vi "2B_Tech_TCP_Packet_TWBOZO_v1.vi"(7 "TCP Packet In":string, 12 "Data Array":string[](array[string])) -> (8 "TCP Binary Packet":string)   [LabVIEW 2014]
panel:
  out "array":string[](array[string])
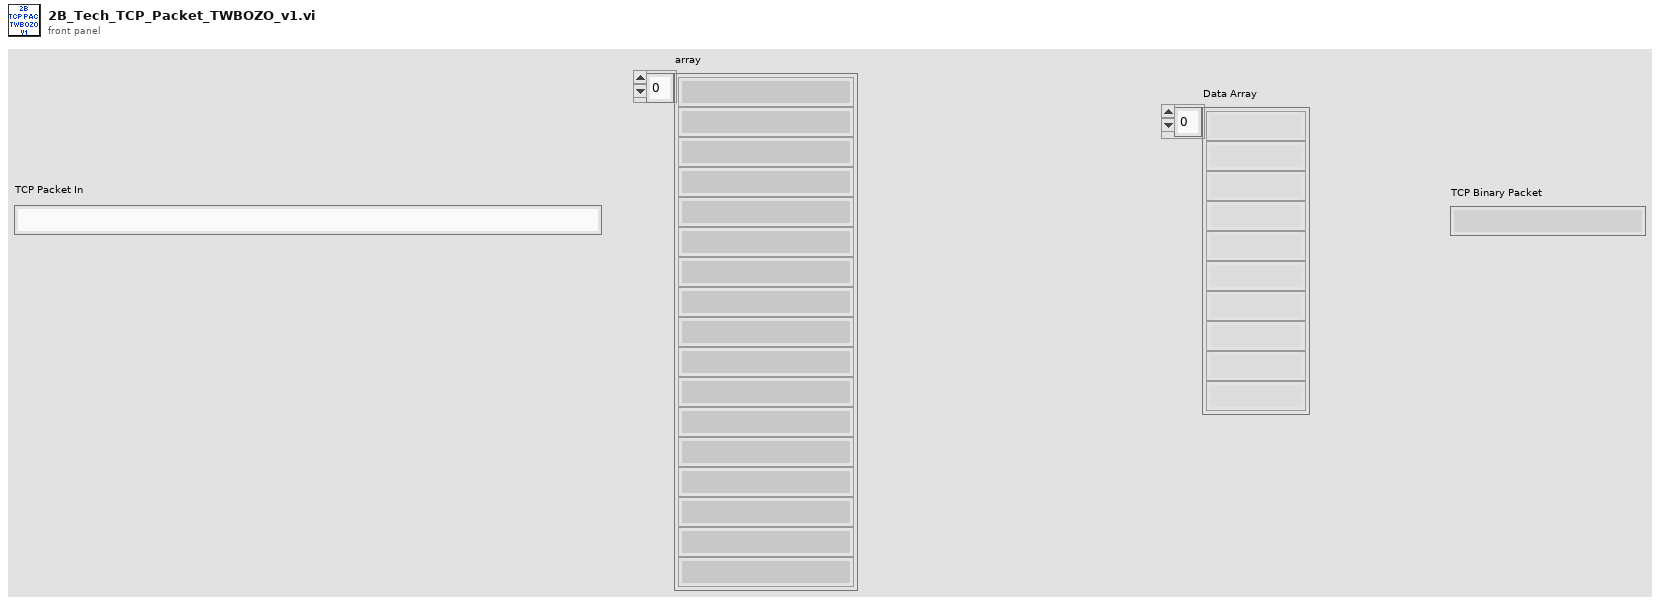
[diagram p1: front panel]
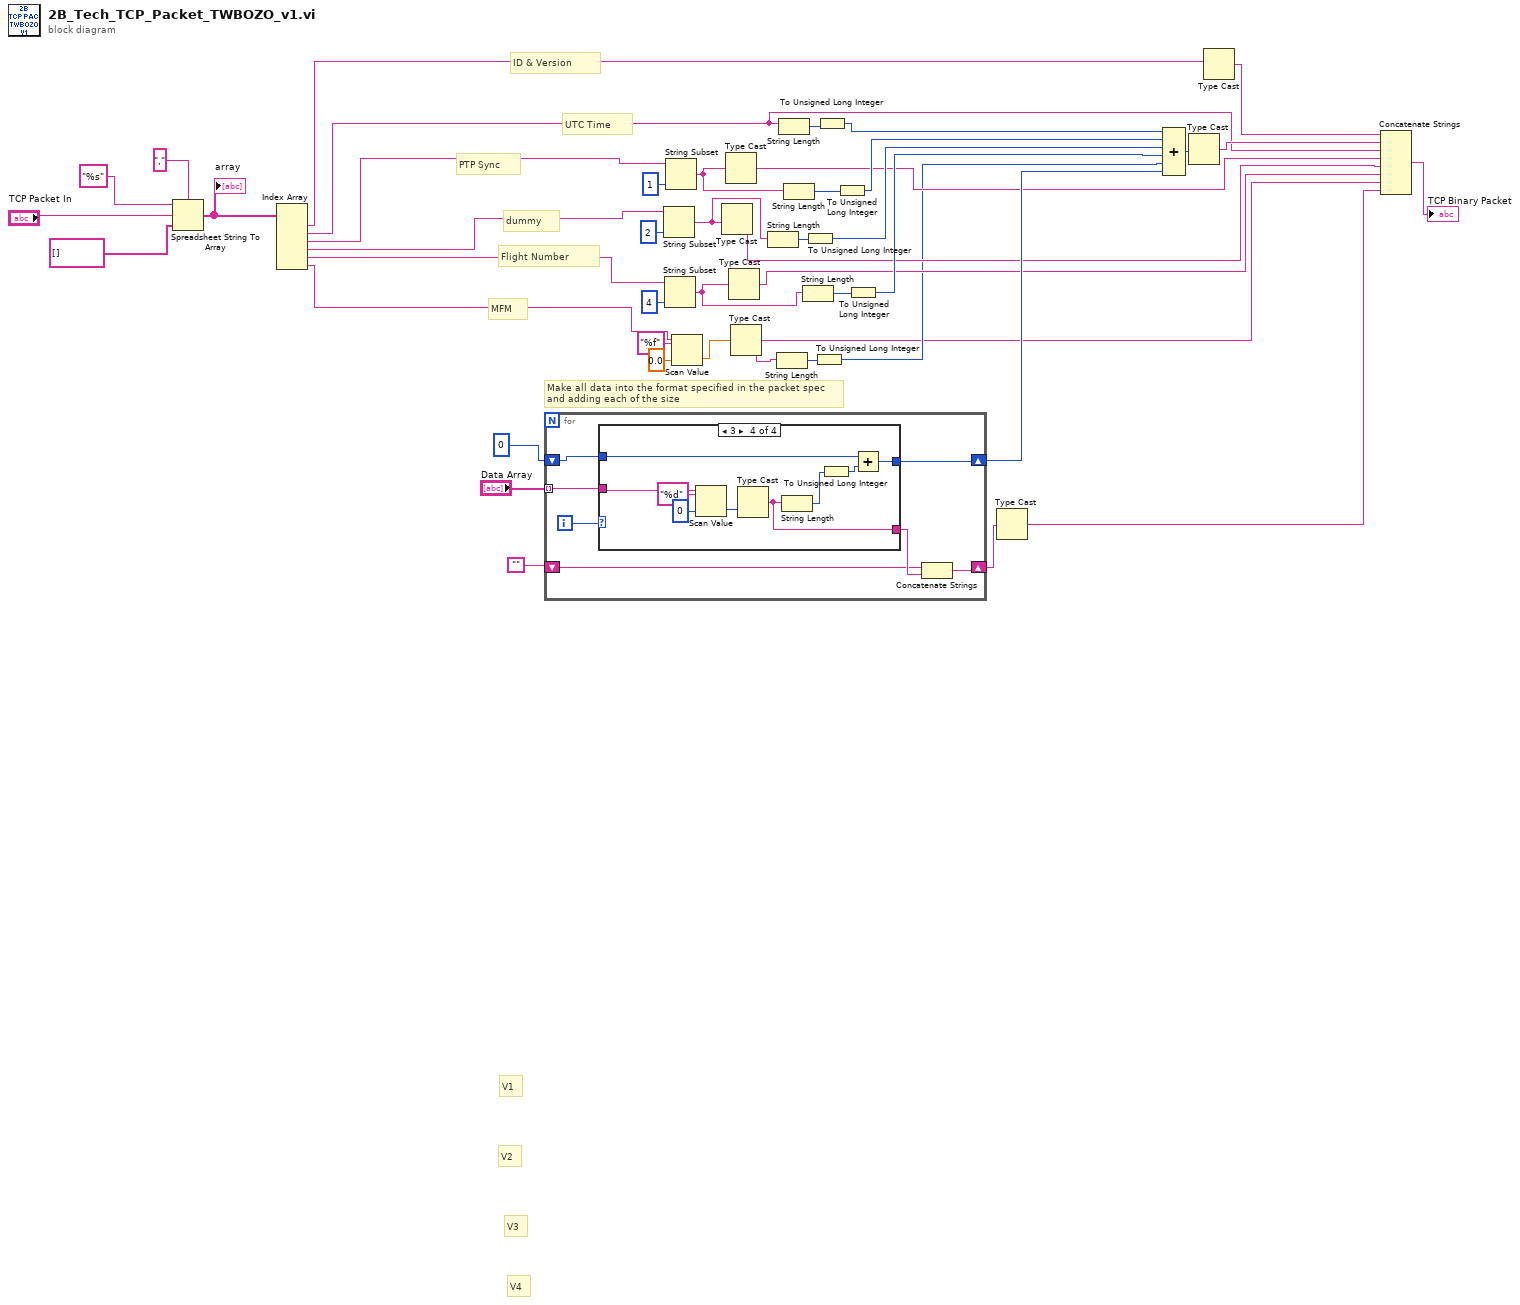
[diagram p0: block diagram]
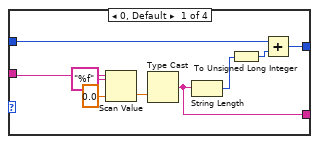
[diagram p2: hidden frame]
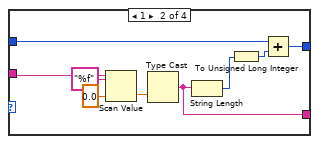
[diagram p3: hidden frame]
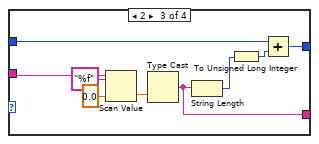
[diagram p4: hidden frame]
diagram:
  # "dummy"
  # "V4"
  # "V3"
  # "V2"
  # "V1"
  # "Flight Number"
  # "MFM"
  # "PTP Sync"
  # "UTC Time"
  # "ID & Version"
  # "Make all data into the format specified in the packet spec\nand adding each of the size"
  n1 = Spreadsheet String To Array(delimiter (Tab)=",", format string="%s", spreadsheet string="TCP Packet In", array type (2D Dbl)=string[] []) -> (array=w16:string[])
  "array" <- w16
  n2 = Index Array(array=w16) -> (element #1=w15:string, element #2=w14:string, element #3=w13:string, element #4=w2:string, element #5=w12:string, element #6=w6:string)  [unwired: 6 in]
  n3 = for {
    tunnel: "Data Array" -> [w50] mode=indexing
    shift-right: [w48] -> w32
    shift-left: u32 0 -> [w49]
    shift-right: [w47] -> w21
    shift-left: "" -> [w45]
    i -> [w51]
    n4 = case shown="3" w51 {
      tunnel: w50 -> [w58 w67 w76 w85]
      tunnel: w49 -> [w56 w65 w74 w83]
      tunnel: [w53 w62 w71 w80] -> w48
      tunnel: [w52 w61 w70 w79] -> w46
      frame 0, Default {
        n5 = Scan Value(string=w58, format string="%f", default (0 dbl)=sgl 0.0 ("default (0 I32)")) -> (value=w60:sgl)  [unwired: 1 out]
        n6 = Type Cast(x=w60) -> (*(type *) &x=w52:string)  [unwired: 1 in]
        n7 = String Length(string=w52) -> (length=w55:i32)
        n8 = To Unsigned Long Integer(number=w55) -> (unsigned 32bit integer=w54:u32)
        n9 = Add(x=w56, y=w54) -> (x+y=w53:u32)
      }
      frame 1 {
        n10 = Scan Value(string=w67, format string="%f", default (0 dbl)=sgl 0.0 ("default (0 I32)")) -> (value=w69:sgl)  [unwired: 1 out]
        n11 = Type Cast(x=w69) -> (*(type *) &x=w61:string)  [unwired: 1 in]
        n12 = String Length(string=w61) -> (length=w64:i32)
        n13 = To Unsigned Long Integer(number=w64) -> (unsigned 32bit integer=w63:u32)
        n14 = Add(x=w65, y=w63) -> (x+y=w62:u32)
      }
      frame 2 {
        n15 = Scan Value(string=w76, format string="%f", default (0 dbl)=sgl 0.0 ("default (0 I32)")) -> (value=w78:sgl)  [unwired: 1 out]
        n16 = Type Cast(x=w78) -> (*(type *) &x=w70:string)  [unwired: 1 in]
        n17 = String Length(string=w70) -> (length=w73:i32)
        n18 = To Unsigned Long Integer(number=w73) -> (unsigned 32bit integer=w72:u32)
        n19 = Add(x=w74, y=w72) -> (x+y=w71:u32)
      }
      frame 3 {
        n20 = Scan Value(string=w85, format string="%d", default (0 dbl)=0 ("default (0 I32)")) -> (value=w87:i32)  [unwired: 1 out]
        n21 = Type Cast(x=w87) -> (*(type *) &x=w79:string)  [unwired: 1 in]
        n22 = String Length(string=w79) -> (length=w82:i32)
        n23 = To Unsigned Long Integer(number=w82) -> (unsigned 32bit integer=w81:u32)
        n24 = Add(x=w83, y=w81) -> (x+y=w80:u32)
      }
    }
    n25 = Concatenate Strings(w45, w46) -> (w47:string)
  }
  n26 = String Subset(string=w2, length (rest)=2 ("length (rest)")) -> (substring=w1:string)  [unwired: 1 in]
  n27 = String Subset(string=w12, length (rest)=4 ("length (rest)")) -> (substring=w25:string)  [unwired: 1 in]
  n28 = String Subset(string=w13, length (rest)=1 ("length (rest)")) -> (substring=w28:string)  [unwired: 1 in]
  n29 = Scan Value(string=w6, format string="%f", default (0 dbl)=sgl 0.0 ("default (0 I32)")) -> (value=w7:sgl)  [unwired: 1 out]
  n30 = Type Cast(x=w1) -> (*(type *) &x=w11:string)  [unwired: 1 in]
  n31 = Type Cast(x=w28) -> (*(type *) &x=w27:string)  [unwired: 1 in]
  n32 = Type Cast(x=w25) -> (*(type *) &x=w26:string)  [unwired: 1 in]
  n33 = Type Cast(x=w7) -> (*(type *) &x=w4:string)  [unwired: 1 in]
  n34 = String Length(string=w1) -> (length=w39:i32)
  n35 = String Length(string=w4) -> (length=w10:i32)
  n36 = String Length(string=w14) -> (length=w44:i32)
  n37 = String Length(string=w28) -> (length=w41:i32)
  n38 = String Length(string=w25) -> (length=w36:i32)
  n39 = To Unsigned Long Integer(number=w39) -> (unsigned 32bit integer=w38:u32)
  n40 = To Unsigned Long Integer(number=w10) -> (unsigned 32bit integer=w5:u32)
  n41 = To Unsigned Long Integer(number=w44) -> (unsigned 32bit integer=w43:u32)
  n42 = To Unsigned Long Integer(number=w41) -> (unsigned 32bit integer=w40:u32)
  n43 = To Unsigned Long Integer(number=w36) -> (unsigned 32bit integer=w35:u32)
  n44 = Type Cast(x=w21) -> (*(type *) &x=w24:string)  [unwired: 1 in]
  n45 = Compound Arithmetic op=ADD(w43, w40, w38, w35, w5, w32) -> (w30:u32)
  n46 = Type Cast(x=w30) -> (*(type *) &x=w29:string)  [unwired: 1 in]
  n47 = Type Cast(x=w15) -> (*(type *) &x=w31:string)  [unwired: 1 in]
  n48 = Concatenate Strings(w31, w29, w14, w27, w11, w26, w4, w24) -> (→"TCP Binary Packet":string)
